vi "Circle_Init.vi"(6 "Radius":dbl, 8 "error in (no error)":errorcluster, 9 "Y":dbl, 10 "X":dbl, 11 "object in":refnum<class "Circle.lvclass">) -> (0 "error out":errorcluster, 3 "object out":refnum<class "Circle.lvclass">)   [LabVIEW 2020, in "Circle.lvclass"]
uses:
  Circle.lvclass
  Circle.lvclass/Circle.ctl
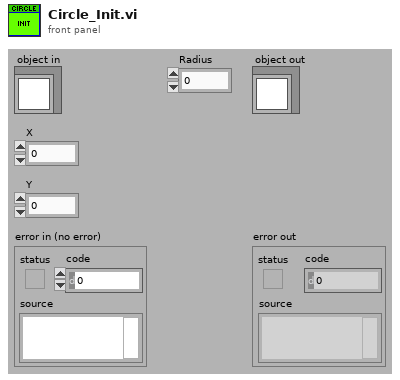
[diagram p1: front panel]
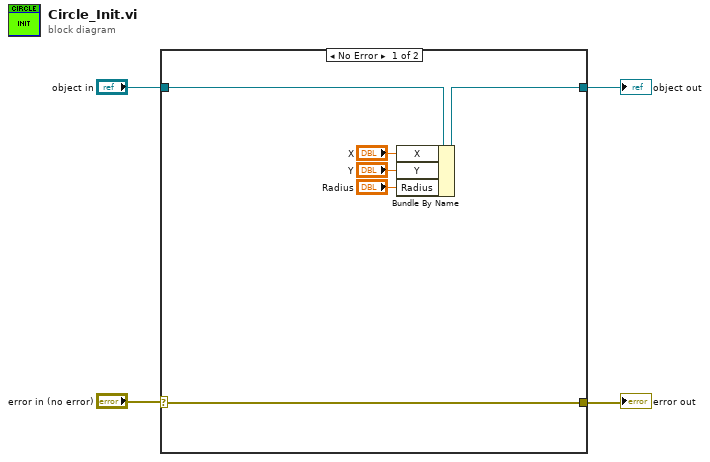
[diagram p0: block diagram]
diagram:
  n1 = case shown="No Error" "error in (no error)" {
    selector: "error in (no error)" -> [w8 w11]
    tunnel: "object in" -> [w10 w12]
    tunnel: [w9 w12] -> w3
    tunnel: [w8 w11] -> w1
    frame No Error {
      n2 = Bundle By Name(cluster=w10, "X"="X", "Y"="Y", "Radius"="Radius") -> (w9:refnum<class "Circle.lvclass">)
    }
    frame Error {
    }
  }
  "object out" <- w3
  "error out" <- w1
